vi "Read termChar.vi"(8 "error in (no error)":errorcluster, 11 "ElectrometerConfiguration in":refnum<class "ElectrometerCOMConfiguration.lvclass">) -> (0 "error out":errorcluster, 2 "termChar":T1, 3 "ElectrometerConfiguration out":refnum<class "ElectrometerCOMConfiguration.lvclass">)   [LabVIEW 2016, in "ElectrometerCOMConfiguration.lvclass"]
uses:
  ElectrometerCOMConfiguration.lvclass
  ts_electrometeruserevents/Typedefs/termChar.ctl
  ElectrometerCOMConfiguration.lvclass/ElectrometerCOMConfiguration.ctl
  ts_electrometeruserevents/Typedefs/ElectrometerTypedefs.lvlib
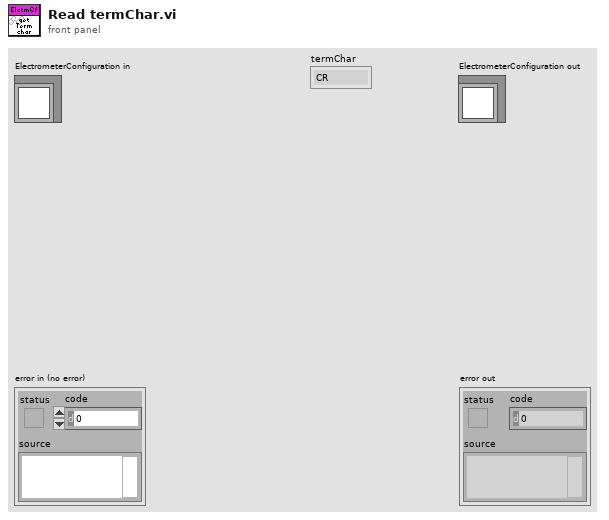
[diagram p1: front panel]
types:
  T1 = typedef "ElectrometerTypedefs.lvlib/termChar.ctl" = enum16{"CR", "CR+LF", "LF", "LF+CR"}
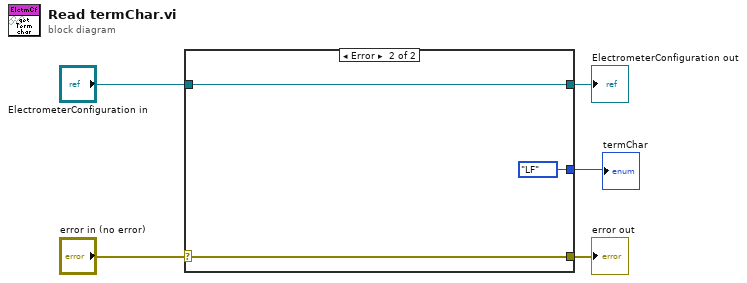
[diagram p0: block diagram]
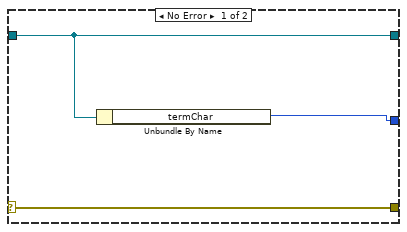
[diagram p2: hidden frame]
diagram:
  n1 = case shown="Error" "error in (no error)" {
    selector: "error in (no error)" -> [w8 w10]
    tunnel: [w8 w10] -> w4
    tunnel: [w7 w11] -> w2
    tunnel: "ElectrometerConfiguration in" -> [w7 w11]
    tunnel: [w6 termChar."LF" ("termChar")] -> w1
    frame No Error {
      n2 = Unbundle By Name(w7) -> ("termChar"=w6:T1)
    }
    frame Error {
    }
  }
  "error out" <- w4
  "ElectrometerConfiguration out" <- w2
  "termChar" <- w1
